vi "PH_O2_Watch.ProcEvents.vi"(0 "i ref in":refnum<vi>, 5 "error in (no error)":errorcluster) -> (14 "i ref out":refnum<vi>, 19 "error out":errorcluster)   [LabVIEW 2014, in "PH_O2_Watch.lvlib"]
doc: "This method is used to define the events the object will listen to. Add your own events here."
uses:
  PH_O2_Watch.lvlib
  CS_Core/BaseProcess/BaseProcess.event definition.ctl
  CS_Core/CAEObj/CAEObj.event definition.ctl
  CS_Core/BaseProcess/BaseProcess.descriptor string definition.ctl
  CS_Core/BaseProcess/BaseProcess.lvlib
  CS_Core/CAEObj/CAEObj.lvlib
  PH_Basics/PH_Common/PH_Common.lvlib
  CS_Core/CSSystem/CSSystemLib/CSSystemLib.lvlib
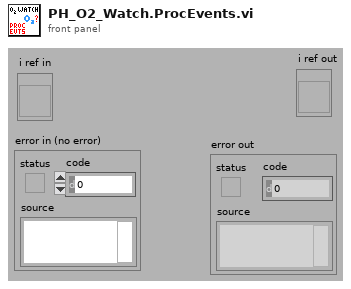
[diagram p1: front panel]
types:
  T1 = typedef "BaseProcess.lvlib/BaseProcess.event definition.ctl" = cluster{"CAEEvtDef":T2, "Data Descriptor":T3}
  T2 = typedef "CAEObj.lvlib/CAEObj.event definition.ctl" = cluster{"URL":string, "enable":bool, "ignoreResID":bool}
  T3 = typedef "BaseProcess.lvlib/BaseProcess.descriptor string definition.ctl" = string
  T4 = typedef "PH_Common.lvlib/PH_DIM.Event Declarer.ctl" = cluster{"Service Name":string, "Selector":string}
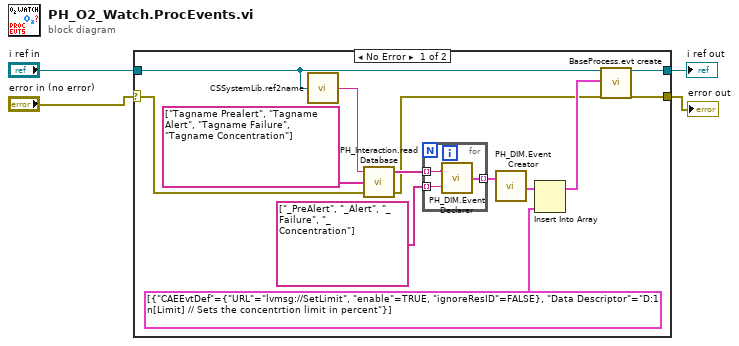
[diagram p0: block diagram]
diagram:
  n1 = case shown="No Error" "error in (no error)" {
    selector: "error in (no error)" -> [w15 w21]
    tunnel: "i ref in" -> [w5 w22]
    tunnel: [w17 w22] -> w3
    tunnel: [w16 w21] -> w2
    frame No Error {
      n2 = call "CSSystemLib.ref2name.vi"("obj refnum"=w5) -> ("name"=w8:string)
      n3 = call "PH_Interaction.read Database.vi"("error in (no error)"=w15, "Strings to search for"=string[] ["Tagname Prealert", "Tagname Alert", "Tagname Failure", "Tagname Concentration"], "DB Entry to read"=w8) -> ("error out"=w6:errorcluster, "Values"=w9:string[])  [unwired: 1 in]
      n4 = for {
        tunnel: [w20] -> w11 mode=indexing
        tunnel: w9 -> [w19] mode=indexing
        tunnel: string[] ["_PreAlert", "_Alert", "_Failure", "_Concentration"] -> [w18] mode=indexing
        n5 = call "PH_DIM.Event Declarer.vi"("Selector"=w18, "Service Name"=w19) -> ("declared DIM Event"=w20:T4)
      }
      n6 = call "PH_DIM.Event Creator.vi"("Trendmessage Services"=w11) -> ("DIM Service Events"=w14:T1[])  [unwired: 18 in]
      n7 = Insert Into Array(array=w14, new element=T1[] [{"CAEEvtDef"={"URL"="lvmsg://SetLimit", "enable"=TRUE, "ignoreResID"=FALSE}, "Data Descriptor"="D:1 n[Limit] // Sets the concentrtion limit in percent"}] ("new events")) -> (w12:T1[])  [unwired: 1 in]
      n8 = call "BaseProcess.evt create.vi"("i ref in"=w5, "newEvents"=w12, "error in (no error)"=w6) -> ("i ref out"=w17:refnum<vi>, "error out"=w16:errorcluster)  [unwired: 13 in, 2 out]
    }
    frame Error {
    }
  }
  "i ref out" <- w3
  "error out" <- w2
